vi "CCVerificationSCU.vi"(7 "remotePort":i32=1234, 8 "error in (no error)":errorcluster, 9 "remoteHost":string="localhost", 10 "remoteAE":string="OFFIS", 11 "clientAETitle":string="Pseudo") -> (0 "error out":errorcluster, 2 "FailureDescription":string, 3 "Result":i32(ring) items=["Failed", "Success", "TimeoutExpired", "Canceled", "AssociationRejected"])   [LabVIEW 2013, in "ClearCanvasLibrary.lvlib"]
uses:
  ClearCanvasLibrary.lvlib
  C:/Users/Simon/SkyDrive/LabView/2013/DM2020/DICOM/ClearCanvasNewBuild/ClearCanvas.Dicom.dll
  ClearCanvasNewBuild/ClearCanvas.Dicom.dll
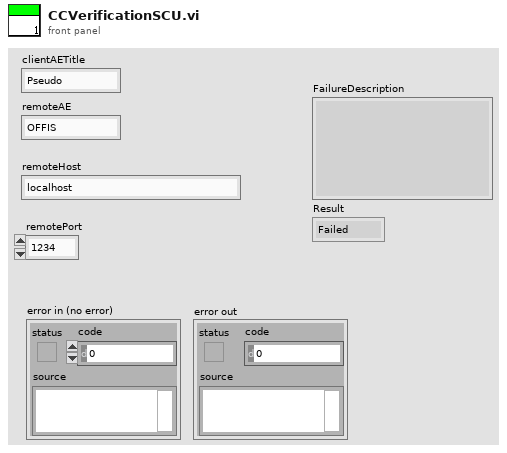
[diagram p1: front panel]
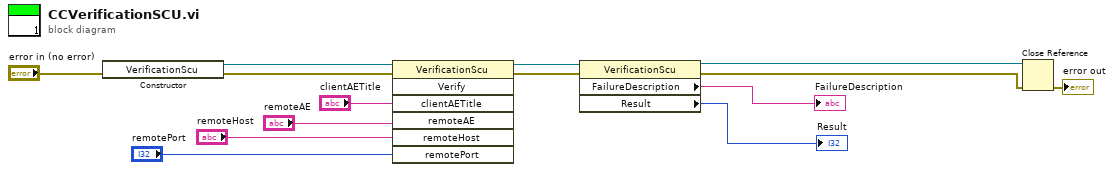
[diagram p0: block diagram]
diagram:
  n1 = constructor class="VerificationScu"(error in="error in (no error)") -> (reference out=w10:refnum<k24>, error out=w9:errorcluster)  [unwired: 2 in, 1 out]
  n2 = invoke class="VerificationScu" method="Verify"(reference=w10, error in=w9, "clientAETitle"="clientAETitle", "remoteAE"="remoteAE", "remoteHost"="remoteHost", "remotePort"="remotePort") -> (reference out=w8:refnum<k24>, error out=w3:errorcluster)  [unwired: 1 in, 5 out]
  n3 = property class="VerificationScu"(reference=w8, error in=w3) -> (reference out=w5:refnum<k24>, error out=w4:errorcluster, "FailureDescription"=→"FailureDescription":string, "Result"=→"Result":i32)
  n4 = Close Reference(reference=w5, error in (no error)=w4) -> (error out=→"error out":errorcluster)
